vi "DSF.Engine.Framework.Get All Transfer Groups.vi"(11 "Framework in":refnum<class "Framework.lvclass">) -> (2 "All Transfer Groups":refnum<class "DSF.Engine.Transfer Group.lvclass">[](array[class]), 3 "Framework out":refnum<class "Framework.lvclass">)   [LabVIEW 2017, in "DSF.Engine.lvlib" / "Framework.lvclass"]
uses:
  Framework.lvclass
  Transfer/DSF.Engine.Transfer Group.lvclass
  Framework.lvclass/Framework.ctl
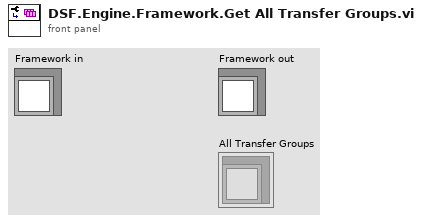
[diagram p1: front panel]
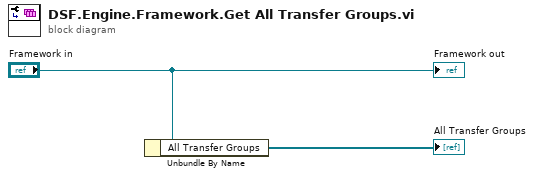
[diagram p0: block diagram]
diagram:
  n1 = Unbundle By Name("Framework in") -> ("All Transfer Groups"=→"All Transfer Groups":refnum<class "DSF.Engine.Transfer Group.lvclass">[])
  "Framework out" <- "Framework in"
